vi "Configure Channel.vi"(8 "error in (no error)":errorcluster, 10 "Channel Setting":T1={"Channel Name (0: Channel 1)"=0, "Coupling (1: DC)"=1, "Vertical Offset (0.0)"=0.0, "Vertical Range (40.0 V)"=40.0, "Probe Attenuation (1.0)"=1.0, "Enable Channel (T: Enable)"=TRUE, "Impedance (0: 1 MOhm)"=0, "Vertical Scale (5.0 V)"=5.0, "Vertical Setting (1: Vertical Range)"=1} {"Vertical Setting (1: Vertical Range)" items=["Vertical Scale", "Vertical Range"]; "Impedance (0: 1 MOhm)" items=["1 MOhm", "50 Ohm"]; "Coupling (1: DC)" items=["AC", "DC"]; "Channel Name (0: Channel 1)" items=["Channel 1", "Channel 2", "Channel 3", "Channel 4"]}, 11 "Abstract in":refnum<class "Abstract.lvclass">) -> (0 "error out":errorcluster, 3 "Abstract out":refnum<class "Abstract.lvclass">)   [LabVIEW 2021, in "Oscilloscope.lvlib" / "Abstract.lvclass"]
uses:
  Abstract.lvclass
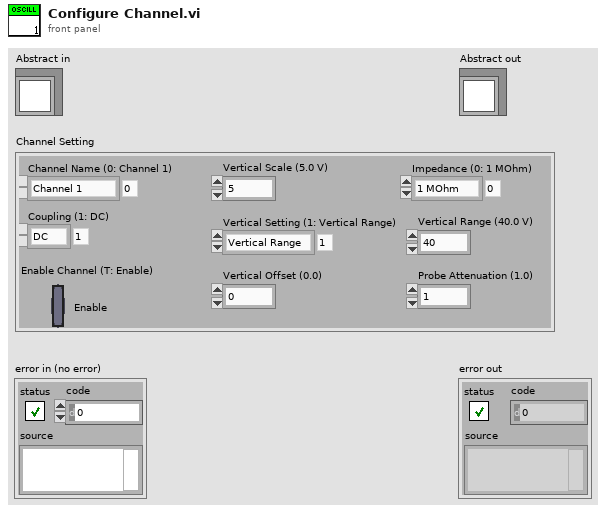
[diagram p1: front panel]
types:
  T1 = cluster{"Channel Name (0: Channel 1)":i32, "Coupling (1: DC)":i32, "Vertical Offset (0.0)":dbl, "Vertical Range (40.0 V)":dbl, "Probe Attenuation (1.0)":dbl, "Enable Channel (T: Enable)":bool, "Impedance (0: 1 MOhm)":i32, "Vertical Scale (5.0 V)":dbl, "Vertical Setting (1: Vertical Range)":i32}
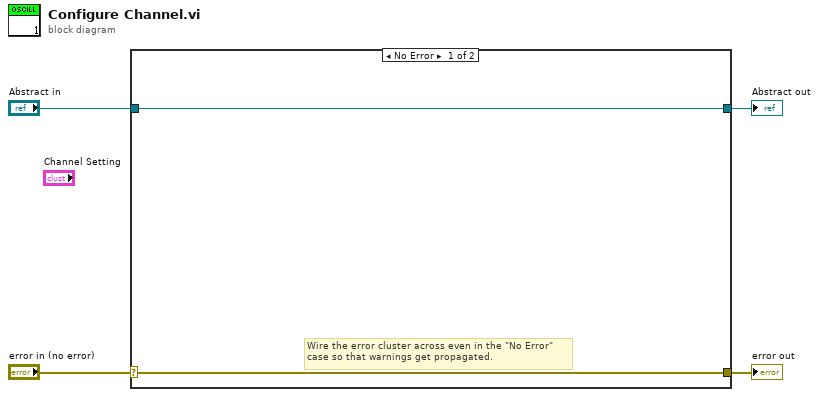
[diagram p0: block diagram]
diagram:
  n1 = case shown="No Error" "error in (no error)" {
    selector: "error in (no error)" -> [w5 w8]
    tunnel: [w5 w8] -> w3
    tunnel: [w6 w7] -> w1
    tunnel: "Abstract in" -> [w6 w7]
    frame No Error {
      # "Wire the error cluster across even in the \"No Error\"\ncase so that warnings get propagated."
    }
    frame Error {
    }
  }
  "error out" <- w3
  "Abstract out" <- w1
